vi "伺服卡配置.vi"() -> ()   [LabVIEW 2013]
uses:
  <vilib>/Utility/config.llb/Write Key (I32).vi
  <vilib>/Utility/config.llb/Read Key (I32).vi
  <vilib>/Utility/config.llb/NI_LVConfig.lvlib
panel:
  out "Array":dbl[](array[numeric])
  in  "油压2":T1(radio)=enum."Boolean"
  in  "电气":T1(radio)=enum."Boolean"
  in  "退出":bool
  in  "油压":T1(radio)=enum."Boolean"
  in  "行程":T1(radio)=enum."Boolean"
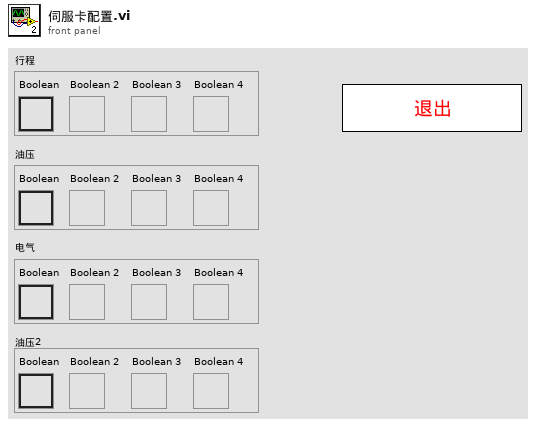
[diagram p1: front panel]
types:
  T1 = enum32{"No Selection", "Boolean", "Boolean 2", "Boolean 3", "Boolean 4"}
  T2 = typedef "NI_LVConfig.lvlib/Config Data RefNum.ctl" = refnum<k1>
  T3 = enum32{"No Selection", "Boolean", "Boolean 2", "Boolean 3", "Boolean 4"}[]
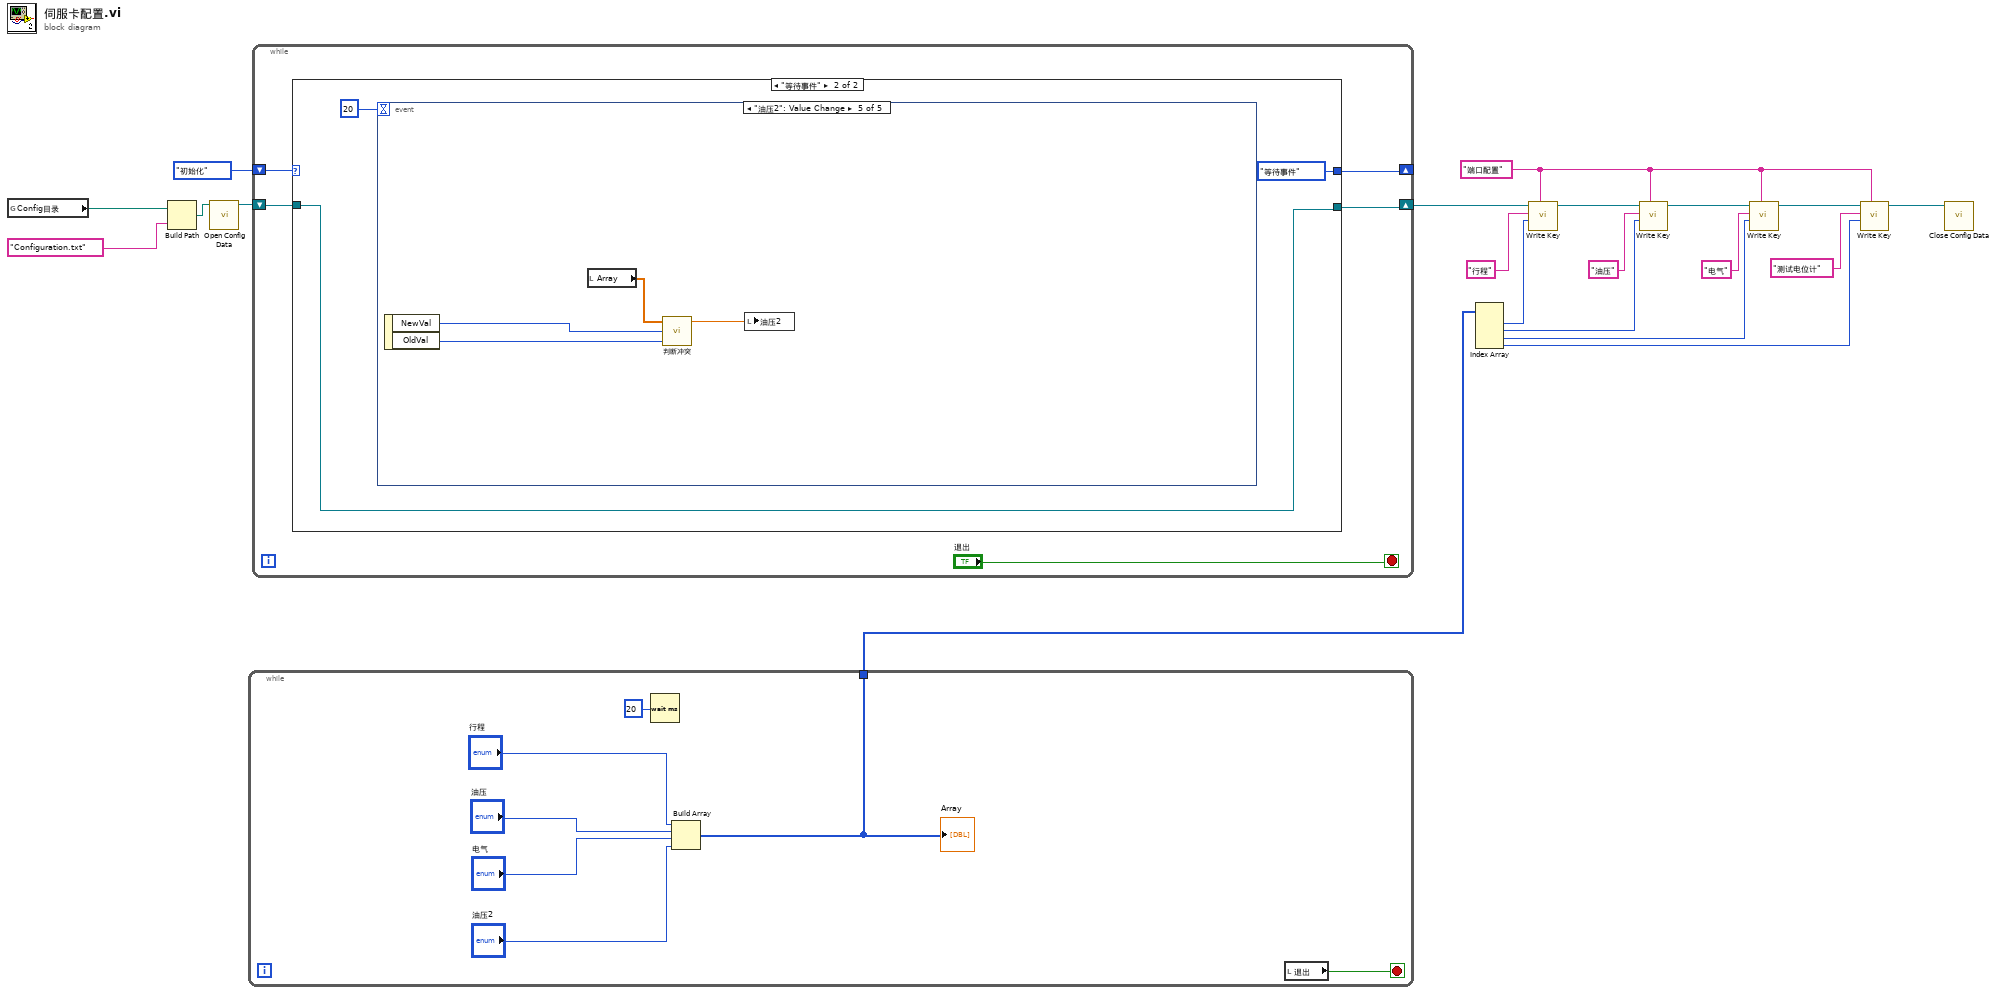
[diagram p0: block diagram]
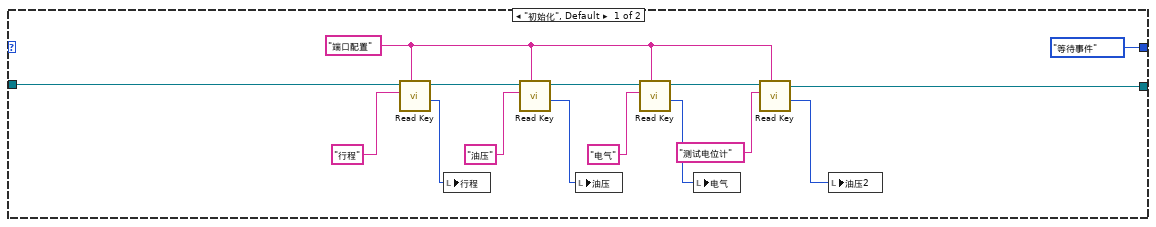
[diagram p2: hidden frame]
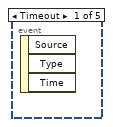
[diagram p3: hidden frame]
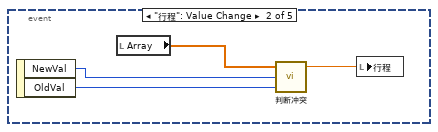
[diagram p4: hidden frame]
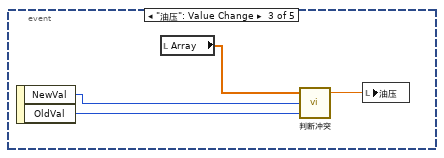
[diagram p5: hidden frame]
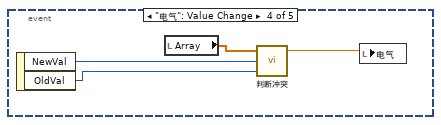
[diagram p6: hidden frame]
diagram:
  w13 = "端口配置" ("Section")
  n1 = global read "Config目录.vi" "Config目录"() -> (w19:path)
  n2 = Build Path(base path=w19, name or relative path="Configuration.txt") -> (appended path=w9:path)
  n3 = call <vilib>:"Open Config Data.vi"("configuration file path"=w9) -> ("refnum"=w8:T2)  [unwired: 8 in, 2 out]
  n4 = while {
    tunnel: [w21] -> w1
    stop <- w22 stop-if-true
    n5 = Wait (ms)(milliseconds to wait=u32 20) -> ()  [unwired: 1 out]
    n6 = Build Array("行程", "油压", "电气", "油压2") -> (w21:T3)
    "Array" <- w21
    n7 = local read "退出"() -> (w22:bool)
  }
  n8 = while {
    shift-right: [w30] -> _
    shift-left: enum16{"初始化", "等待事件"}."初始化" -> [w32]
    shift-right: [w28] -> w7
    shift-left: w8 -> [w29]
    stop <- "退出" stop-if-true
    n9 = case shown="\"等待事件\"" w32 {
      tunnel: [enum16{"初始化", "等待事件"}."等待事件" enum16{"初始化", "等待事件"}."等待事件"] -> w30
      tunnel: w29 -> [w33 w48]
      tunnel: [w34 w48] -> w28
      frame "初始化", Default {
        w42 = "端口配置" ("Section")
        n10 = call-poly <vilib>:"Read Key.vi"("section"=w42, "key"="行程" ("Key"), "refnum"=w33) -> ("value"=w46:i32, "refnum out"=w45:T2)  [unwired: 5 in, 2 out]
        n11 = local write "行程"(w46) -> ()
        n12 = call-poly <vilib>:"Read Key.vi"("section"=w42, "key"="油压" ("Key"), "refnum"=w45) -> ("value"=w40:i32, "refnum out"=w44:T2)  [unwired: 5 in, 2 out]
        n13 = local write "油压"(w40) -> ()
        n14 = call-poly <vilib>:"Read Key.vi"("section"=w42, "key"="电气" ("Key"), "refnum"=w44) -> ("value"=w35:i32, "refnum out"=w43:T2)  [unwired: 5 in, 2 out]
        n15 = local write "电气"(w35) -> ()
        n16 = call-poly <vilib>:"Read Key.vi"("section"=w42, "key"="测试电位计" ("Key"), "refnum"=w43) -> ("value"=w36:i32, "refnum out"=w34:T2)  [unwired: 5 in, 2 out]
        n17 = local write "油压2"(w36) -> ()
      }
      frame "等待事件" {
        n18 = event shown="[4] \"油压2\": Value Change" {
          selector: _ -> [_ _ _ _ _]
          dyn-events: _ -> [_ _ _ _ _]
          timeout: 20 -> [_ _ _ _ _]
          event Timeout {
            n19 = event-data() -> ()  [unwired: 1 in, 3 out]
          }
          event "行程": Value Change {
            n20 = event-data() -> ("NewVal"=w53:T1, "OldVal"=w52:T1)  [unwired: 1 in]
            n21 = local read "Array"() -> (w54:dbl[])
            n22 = call "判断冲突.vi"("OldVal"=w52, "NewVal"=w53, "Array"=w54) -> ("OutVal"=w51:dbl)  [unwired: 2 in]
            n23 = local write "行程"(w51) -> ()
          }
          event "油压": Value Change {
            n24 = event-data() -> ("NewVal"=w57:T1, "OldVal"=w58:T1)  [unwired: 1 in]
            n25 = local read "Array"() -> (w56:dbl[])
            n26 = call "判断冲突.vi"("OldVal"=w58, "NewVal"=w57, "Array"=w56) -> ("OutVal"=w55:dbl)  [unwired: 2 in]
            n27 = local write "油压"(w55) -> ()
          }
          event "电气": Value Change {
            n28 = event-data() -> ("NewVal"=w59:T1, "OldVal"=w60:T1)  [unwired: 1 in]
            n29 = local read "Array"() -> (w61:dbl[])
            n30 = call "判断冲突.vi"("OldVal"=w60, "NewVal"=w59, "Array"=w61) -> ("OutVal"=w62:dbl)  [unwired: 2 in]
            n31 = local write "电气"(w62) -> ()
          }
          event "油压2": Value Change {
            n32 = event-data() -> ("NewVal"=w64:T1, "OldVal"=w65:T1)  [unwired: 1 in]
            n33 = local read "Array"() -> (w63:dbl[])
            n34 = call "判断冲突.vi"("OldVal"=w65, "NewVal"=w64, "Array"=w63) -> ("OutVal"=w66:dbl)  [unwired: 2 in]
            n35 = local write "油压2"(w66) -> ()
          }
        }
      }
    }
  }
  n36 = Index Array(array=w1) -> (element #1=w5:T1, element #2=w4:T1, element #3=w3:T1, element #4=w2:T1)  [unwired: 4 in]
  n37 = call-poly <vilib>:"Write Key.vi"("section"=w13, "value"=w5, "key"="行程" ("Key"), "refnum"=w7) -> ("refnum out"=w16:T2)  [unwired: 5 in, 2 out]
  n38 = call-poly <vilib>:"Write Key.vi"("section"=w13, "value"=w4, "key"="油压" ("Key"), "refnum"=w16) -> ("refnum out"=w15:T2)  [unwired: 5 in, 2 out]
  n39 = call-poly <vilib>:"Write Key.vi"("section"=w13, "value"=w3, "key"="电气" ("Key"), "refnum"=w15) -> ("refnum out"=w14:T2)  [unwired: 5 in, 2 out]
  n40 = call-poly <vilib>:"Write Key.vi"("section"=w13, "value"=w2, "key"="测试电位计" ("Key"), "refnum"=w14) -> ("refnum out"=w6:T2)  [unwired: 5 in, 2 out]
  n41 = call <vilib>:"Close Config Data.vi"("refnum"=w6) -> ()  [unwired: 9 in, 2 out]
